vi "Dot Product.vi"   [LabVIEW 2014, in "NI_AALBase.lvlib"]
doc: "Computes the dot product of <B>X Vector</B> and <B>Y Vector</B>. The data types you wire to the <B>X Vector</B> and <B>Y Vector</B> inputs determine the polymorphic instance to use."
uses:
  NI_AALBase.lvlib
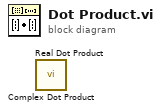
[diagram p0: block diagram]
diagram:
  n1 = call "Complex Dot Product.vi"() -> ()  [unwired: 2 in, 2 out]
  n2 = call "Real Dot Product.vi"() -> ()  [unwired: 2 in, 2 out]
